vi "SDO_DRIVE_MODULE_ACQUIRE.vi"(6 "Pass_Through_Time":dbl=-1.0 format="%33.4f", 7 "Swerve Module Inx":i32, 11 "Swerve Module TypDef":T4[](array[typedef])) -> (1 "SWERVE DRIVE MODULE POSITION":T1={"Distance"=0.0, "Angle"={"VALUE"=0.0, "COS"=1.0, "SIN"=0.0}, "P"=FALSE} {"Angle"."SIN" format="%13.4f"; "Angle"."COS" format="%13.4f"; "Angle"."VALUE" format="%13.4f"}, 3 "Swerve Module State":T3={"Speed"=0.0, "Angle"={"VALUE"=0.0, "COS"=1.0, "SIN"=0.0}} {"Angle"."SIN" format="%13.4f"; "Angle"."COS" format="%13.4f"; "Angle"."VALUE" format="%13.4f"})   [LabVIEW 2019]
uses:
  SDO_DRIVE_MODULE_TYPDEF.ctl
  <vilib>/Rock Robotics/WPI/MotorControl/WPI_MotorControlDeviceRef.ctl
  <vilib>/Rock Robotics/WPI/MotorControl/WPI_MotorControlType.ctl
  <vilib>/Rock Robotics/SystemInterfaces/DIO/FPGA_DIOPWMChannel.ctl
  <vilib>/Rock Robotics/WPI/PWM/WPI_PWMDeadband.ctl
  <vilib>/Rock Robotics/SystemInterfaces/DIO/FPGA_DIOChannel.ctl
  <vilib>/Rock Robotics/WPI/Encoder/WPI_EncoderDevRef.ctl
  <vilib>/Rock Robotics/SystemInterfaces/Encoder/FPGA_EncoderIdx.ctl
  <vilib>/Rock Robotics/SystemInterfaces/Counter/FPGA_CounterCtrSystemIndex.ctl
  <vilib>/Rock Robotics/WPI/Encoder/WPI_EncoderType.ctl
  <vilib>/Rock Robotics/WPI/ThirdParty/JAS_Junk/TrajLib/TypeDef/SWERVE_DRIVE_MODULE_STATE.ctl
  <vilib>/Rock Robotics/WPI/ThirdParty/JAS_Junk/TrajLib/TypeDef/ROTATION2D.ctl
  <vilib>/Rock Robotics/WPI/ThirdParty/JAS_Junk/TrajLib/TypeDef/SWERVE_DRIVE_MODULE_POSITION.ctl
  <vilib>/Rock Robotics/WPI/ThirdParty/JAS_Junk/TrajLib/VI/Util_GetTime_U32.vi
  <vilib>/Rock Robotics/WPI/ThirdParty/JAS_Junk/TrajLib/MathUtil_InputModulus.vi
  <vilib>/Rock Robotics/WPI/ThirdParty/JAS_Junk/TrajLib/VI/Util_GetTime_U64.vi
  <vilib>/Rock Robotics/WPI/ThirdParty/JAS_Junk/TrajLib/Trajectory_Library.lvlib
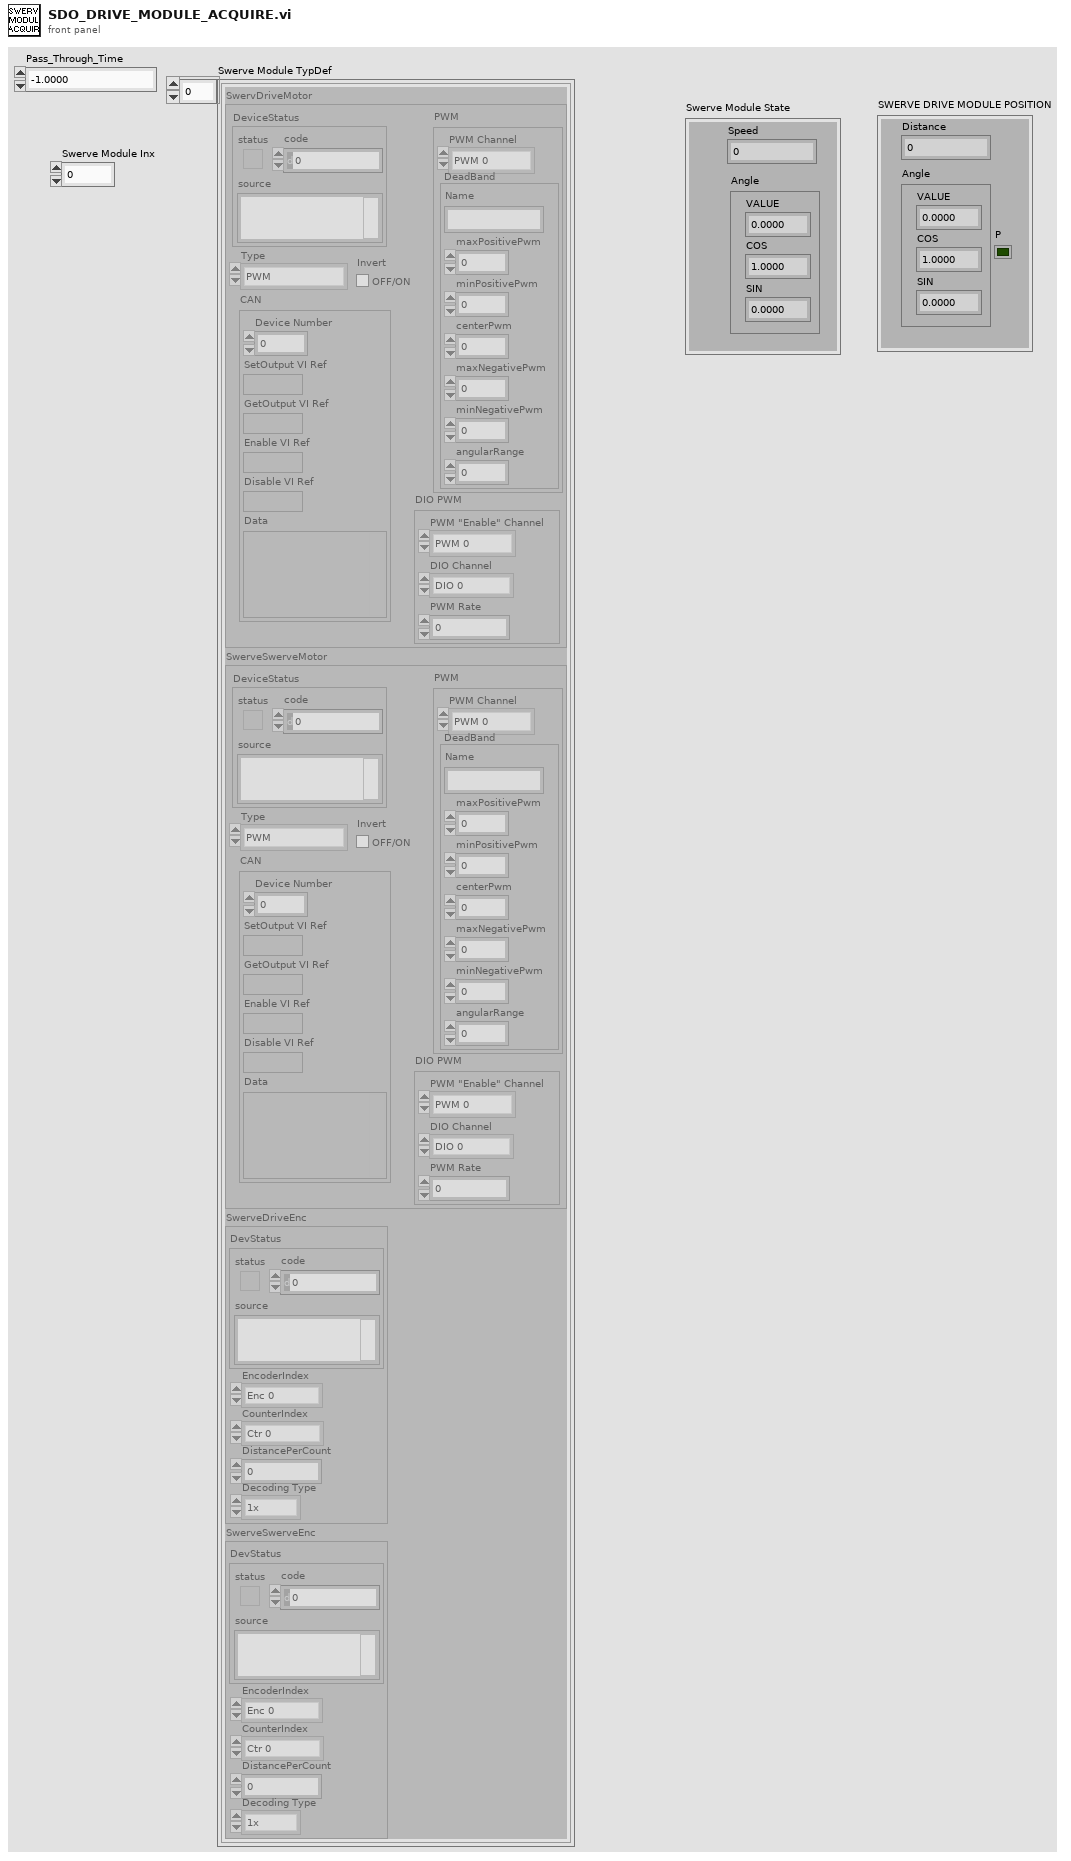
[diagram p1: front panel]
types:
  T1 = typedef "Trajectory_Library.lvlib/SWERVE_DRIVE_MODULE_POSITION.ctl" = cluster{"Distance":dbl, "Angle":T2, "P":bool}
  T2 = typedef "Trajectory_Library.lvlib/ROTATION2D.ctl" = cluster{"VALUE":dbl, "COS":dbl, "SIN":dbl}
  T3 = typedef "Trajectory_Library.lvlib/SWERVE_DRIVE_MODULE_STATE.ctl" = cluster{"Speed":dbl, "Angle":T2}
  T4 = typedef "SDO_DRIVE_MODULE_TYPDEF.ctl" = cluster{"SwervDriveMotor":T5, "SwerveSwerveMotor":T5, "SwerveDriveEnc":T10, "SwerveSwerveEnc":T10}
  T5 = typedef "WPI_MotorControlDeviceRef.ctl" = cluster{"DeviceStatus":errorcluster, "Type":T6, "PWM":cluster{"PWM Channel":T7, "DeadBand":T8}, "CAN":cluster{"Device Number":u8, "SetOutput VI Ref":variant, "GetOutput VI Ref":variant, "Enable VI Ref":variant, "Disable VI Ref":variant, "Data":variant}, "Invert":bool, "DIO PWM":cluster{"PWM \"Enable\" Channel":T7, "DIOChannel":T9, "PWM Rate":dbl}}
  T6 = typedef "WPI_MotorControlType.ctl" = enum16{"PWM", "CAN", "DIO PWM"}
  T7 = typedef "FPGA_DIOPWMChannel.ctl" = enum8{"PWM 0", "PWM 1", "PWM 2", "PWM 3", "PWM 4", "PWM 5", "PWM 6", "PWM 7", "PWM 8", "PWM 9", "PWM MXP 0", "PWM MXP 1", "PWM MXP 2", "PWM MXP 3", "PWM MXP 4", "PWM MXP 5", "PWM MXP 6", "PWM MXP 7", "PWM MXP 8", "PWM MXP 9", "Invalid"}
  T8 = typedef "WPI_PWMDeadband.ctl" = cluster{"Name":string, "maxPositivePwm":i32, "minPositivePwm":i32, "centerPwm":i32, "maxNegativePwm":i32, "minNegativePwm":i32, "angularRange":u16}
  T9 = typedef "FPGA_DIOChannel.ctl" = enum8{"DIO 0", "DIO 1", "DIO 2", "DIO 3", "DIO 4", "DIO 5", "DIO 6", "DIO 7", "DIO 8", "DIO 9", "DIO MXP 0", "DIO MXP 1", "DIO MXP 2", "DIO MXP 3", "DIO MXP 4", "DIO MXP 5", "DIO MXP 6", "DIO MXP 7", "DIO MXP 8", "DIO MXP 9", "DIO MXP 10", "DIO MXP 11", "DIO MXP 12", "DIO MXP 13", "DIO MXP 14", "DIO MXP 15", "SPI Port CS1", "SPI Port CS2", "SPI Port CS3", "SPI Port MISO", "SPI Port MOSI", "Invalid"}
  T10 = typedef "WPI_EncoderDevRef.ctl" = cluster{"DevStatus":errorcluster, "EncoderIndex":T11, "CounterIndex":T12, "DistancePerCount":dbl, "Decoding Type":T13}
  T11 = typedef "FPGA_EncoderIdx.ctl" = enum8{"Enc 0", "Enc 1", "Enc 2", "Enc 3", "Enc 4", "Enc 5", "Enc 6", "Enc 7", "Invalid"}
  T12 = typedef "FPGA_CounterCtrSystemIndex.ctl" = enum8{"Ctr 0", "Ctr 1", "Ctr 2", "Ctr 3", "Ctr 4", "Ctr 5", "Ctr 6", "Ctr 7", "Invalid"}
  T13 = typedef "WPI_EncoderType.ctl" = enum16{"1x", "2x", "4x"}
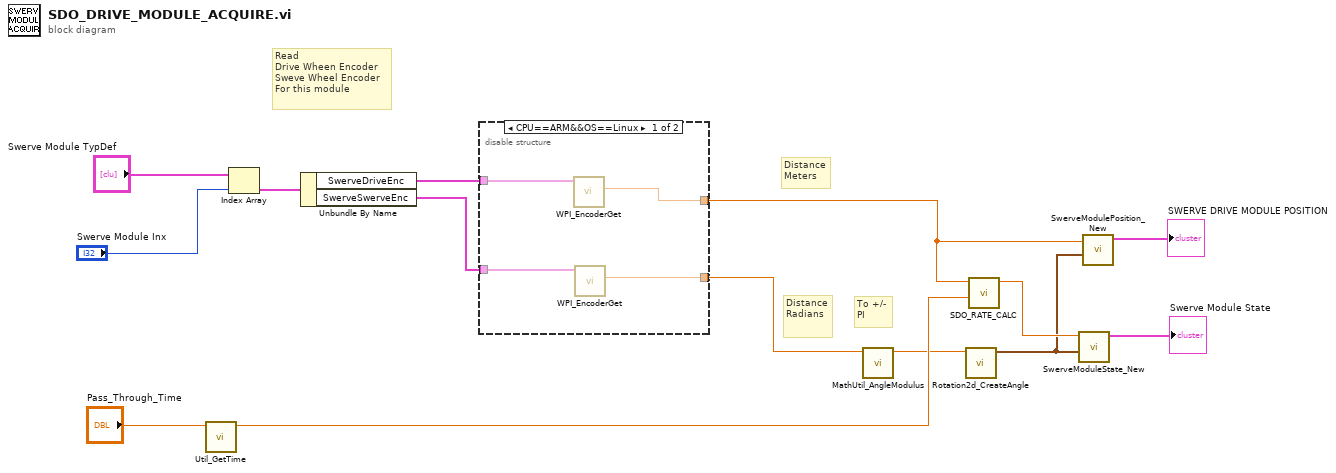
[diagram p0: block diagram]
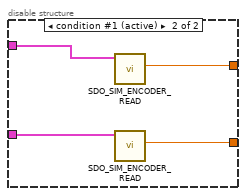
[diagram p2: hidden frame]
diagram:
  # "Read \nDrive Wheen Encoder\nSweve Wheel Encoder\nFor this module"
  # "Distance\nRadians"
  # "Distance\nMeters"
  # "To +/-\nPI"
  n1 = call <vilib>:"Util_GetTime.vi"("Pass_Through_Time"="Pass_Through_Time") -> ("FPGA_Time_Seconds"=w9:dbl)  [unwired: 8 in, 2 out]
  n2 = Index Array(array="Swerve Module TypDef", index="Swerve Module Inx") -> (element=w5:T4)
  n3 = Unbundle By Name(w5) -> ("SwerveDriveEnc"=w4:T10, "SwerveSwerveEnc"=w1:T10)
  n4 = disable-structure shown="CPU==ARM&&OS==Linux" {
    disable-tunnel: w4 -> [w18 w22]
    disable-tunnel: [w16 w21] -> w3
    disable-tunnel: w1 -> [w17 w20]
    disable-tunnel: [w15 w19] -> w2
    frame condition #0 {
      n5 = call <vilib>:"WPI_EncoderGet.vi"("EncoderDevRef"=w18) -> ("Distance"=w16:dbl)  [unwired: 5 in, 5 out]
      n6 = call <vilib>:"WPI_EncoderGet.vi"("EncoderDevRef"=w17) -> ("Distance"=w15:dbl)  [unwired: 5 in, 5 out]
    }
    frame condition #1 (active) {
      n7 = call "SDO_SIM_ENCODER_READ.vi"("EncoderReference"=w22) -> ("Distance"=w21:dbl)  [unwired: 9 in, 1 out]
      n8 = call "SDO_SIM_ENCODER_READ.vi"("EncoderReference"=w20) -> ("Distance"=w19:dbl)  [unwired: 9 in, 1 out]
    }
  }
  n9 = call <vilib>:"MathUtil_AngleModulus.vi"("InputAngle"=w2) -> ("ModulsAngle"=w8:dbl)  [unwired: 10 in]
  n10 = call <vilib>:"Rotation2d_CreateAngle.vi"("Angle"=w8) -> ("ROTATION"=w12:T2)  [unwired: 10 in]
  n11 = call "SDO_RATE_CALC.vi"("Time"=w9, "Input"=w3) -> ("Output"=w13:dbl)  [unwired: 9 in]
  n12 = call <vilib>:"SwerveModuleState_New.vi"("ROTATION"=w12, "Speed"=w13) -> ("SWERVE_DRIVE_MODULE_STATE"=→"Swerve Module State":T3)  [unwired: 9 in]
  n13 = call <vilib>:"SwerveModulePosition_New.vi"("ROTATION"=w12, "Distance"=w3) -> ("SWERVE_DRIVE_MODULE_POSITION"=→"SWERVE DRIVE MODULE POSITION":T1)  [unwired: 9 in]
